vi "ACT_Loop.vi"() -> ()   [LabVIEW 2023, in "2024 Elevator_ACT.lvlib"]
uses:
  2024 Elevator_ACT.lvlib
  Cluster_CMD_ACT_Data.ctl
  <vilib>/Rock Robotics/WPI/Solenoid/WPI_SolenoidValue.ctl
  ENUM_ACT_State.ctl
  <vilib>/Rock Robotics/WPI/Compressor/WPI_CompressorDevRef.ctl
  <vilib>/Rock Robotics/WPI/Solenoid/WPI_SolenoidChannel.ctl
  <vilib>/Rock Robotics/WPI/Solenoid/WPI_SolenoidDevRef.ctl
  ENUM_ACT_Action.ctl
  <vilib>/Rock Robotics/WPI/Compressor/WPI_CompressorFeedbackMode.ctl
  <vilib>/Rock Robotics/WPI/Solenoid/WPI_SolenoidOpenDouble.vi
  RoboRIO Utilities/Global_STOP.vi
  Global_CMD_ACT_Data In.vi
  <vilib>/Rock Robotics/WPI/Solenoid/WPI_SolenoidSetEnum.vi
  Global_ACT_Data Out.vi
panel:
  out "Lift Output":T1
  out "Comp Enabled":bool
  out "Comp Running":bool
  out "Input DBL Data":T2
  out "Output DBL Data":dbl
  out "Cycle Time (S)":dbl format="%.3g"
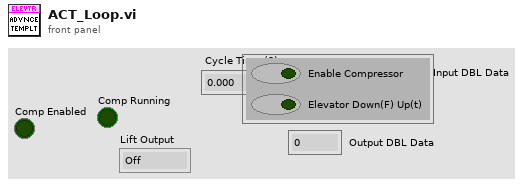
[diagram p1: front panel]
types:
  T1 = typedef "WPI_SolenoidValue.ctl" = enum16{"Off", "On", "Forward", "Reverse"}
  T2 = typedef "2024 Elevator_ACT.lvlib/Cluster_CMD_ACT_Data.ctl" = cluster{"Enable Compressor":bool, "Elevator Down(F) Up(t)":bool}
  T3 = typedef "WPI_SolenoidDevRef.ctl" = cluster{"DevStatus":errorcluster, "Pneumatics Control Module":u8, "Forward Solenoid Channel":T4, "Reverse Solenoid Channel":T4}
  T4 = typedef "WPI_SolenoidChannel.ctl" = enum8{"Solenoid 0", "Solenoid 1", "Solenoid 2", "Solenoid 3", "Solenoid 4", "Solenoid 5", "Solenoid 6", "Solenoid 7", "Solenoid 8", "Solenoid 9", "Solenoid 10", "Solenoid 11", "Solenoid 12", "Solenoid 13", "Solenoid 14", "Solenoid 15", "Invalid"}
  T5 = typedef "WPI_CompressorDevRef.ctl" = cluster{"DevStatus":errorcluster, "Pneumatics Control Module":u8}
  T6 = typedef "2024 Elevator_ACT.lvlib/ENUM_ACT_State.ctl" = enum16{"Startup", "Compressing", "NOT Compressing", "Shutdown"}
  T7 = cluster{"CompressorDevRef":T5, "State":T6, "Previous State":T6, "Current Time":timestamp, "Previous Time":timestamp, "Start Time":timestamp, "Target Time (ms)":u32, "Cycle Time(S)":dbl, "ACT Input":T2, "ACT Output DBL":dbl, "Elevator Ref":T3, "Previous CMD Elevator":bool, "ELEVATOR change":bool, "Comp Enabled":bool, "Comp Running":bool, "Lift Output":T1}
  T8 = typedef "WPI_CompressorFeedbackMode.ctl" = enum16{"Analog Only", "Digital Only", "Hybrid"}
  T9 = cluster{"Feedback Sensor":T8, "Max Pressure (PSI)":dbl, "Min Pressure (PSI)":dbl}
  T10 = typedef "2024 Elevator_ACT.lvlib/ENUM_ACT_Action.ctl" = enum16{"No Action", "Reset Time", "Reset All", "Start Compressor", "Stop Compressor", "Lift Solenoid", "Lower Solenoid", "OFF Solenoid"}
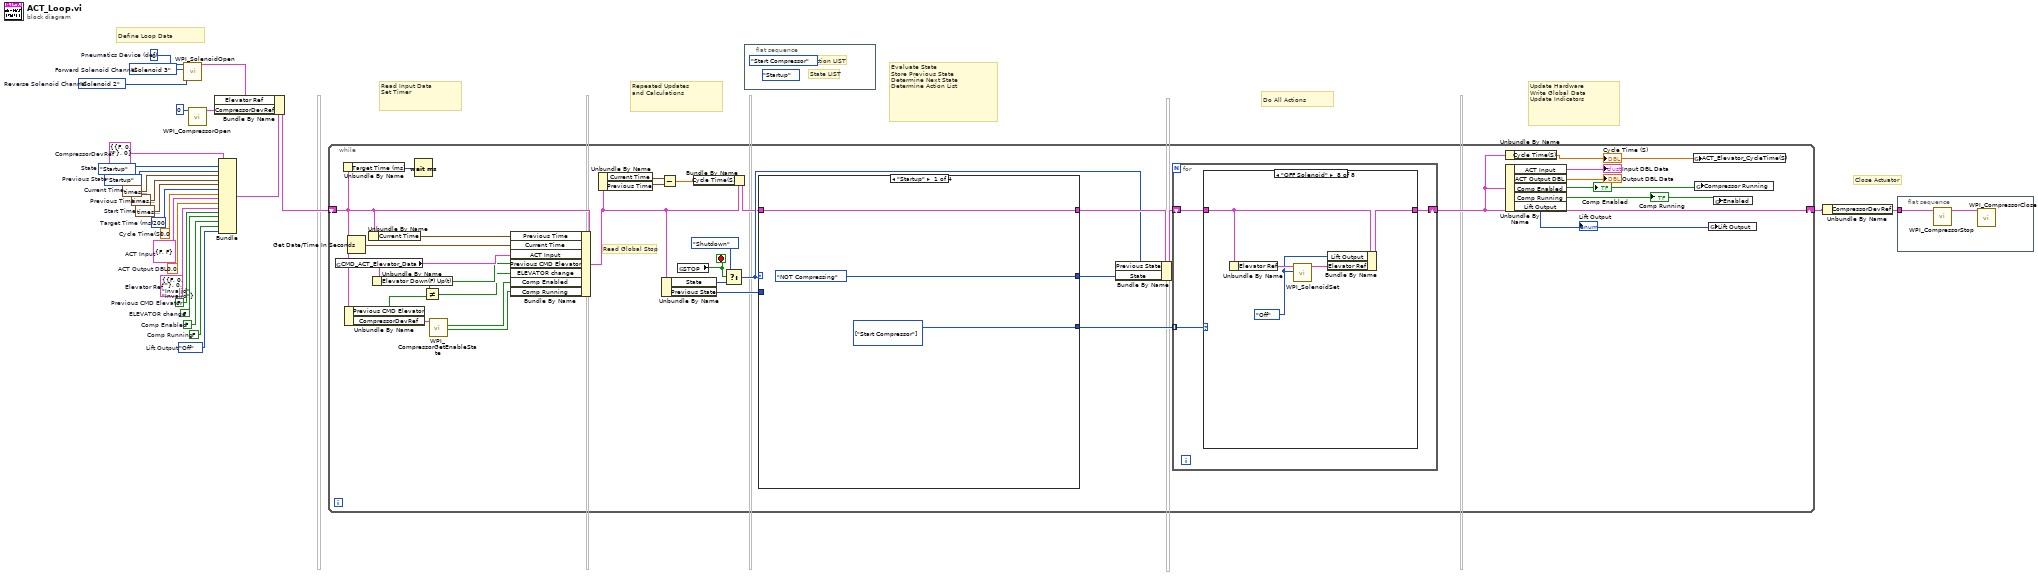
[diagram p0: block diagram]
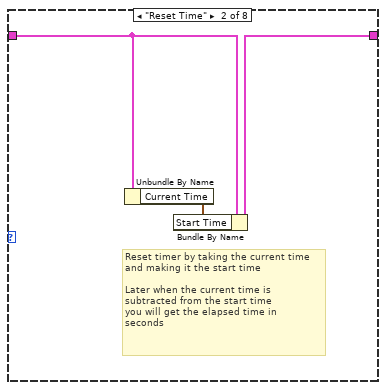
[diagram p3: hidden frame]
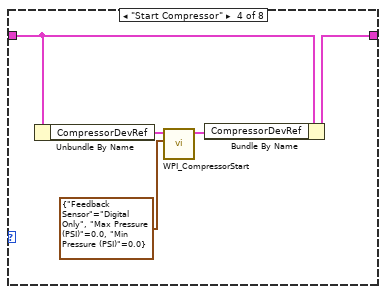
[diagram p5: hidden frame]
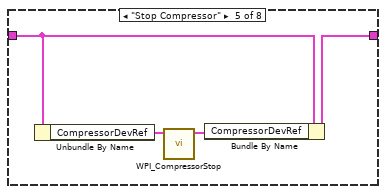
[diagram p6: hidden frame]
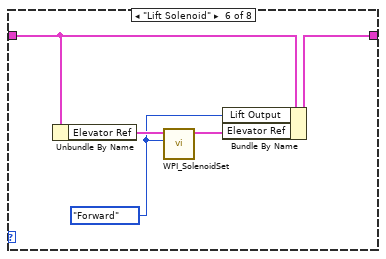
[diagram p7: hidden frame]
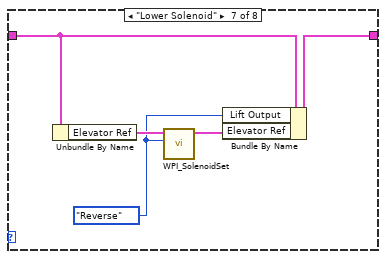
[diagram p8: hidden frame]
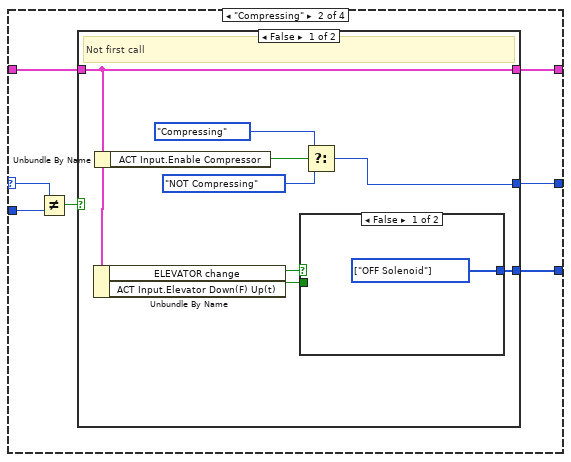
[diagram p9: hidden frame]
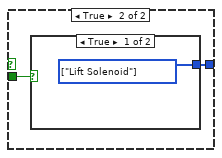
[diagram p10: hidden frame]
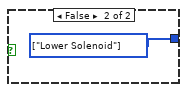
[diagram p11: hidden frame]
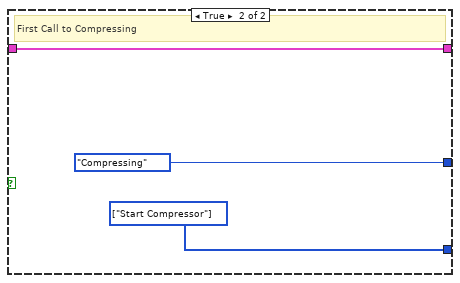
[diagram p12: hidden frame]
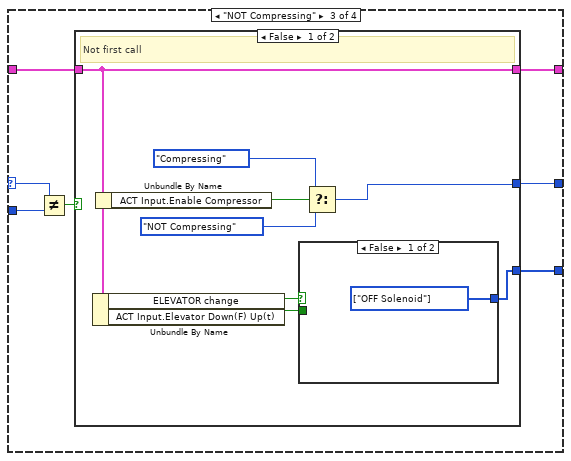
[diagram p13: hidden frame]
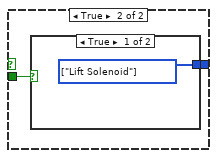
[diagram p14: hidden frame]
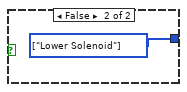
[diagram p15: hidden frame]
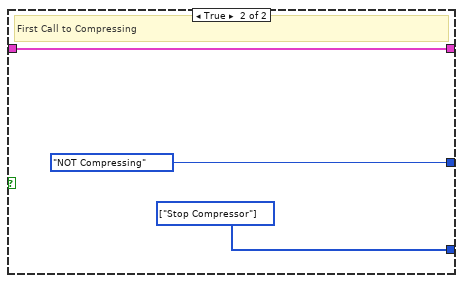
[diagram p16: hidden frame]
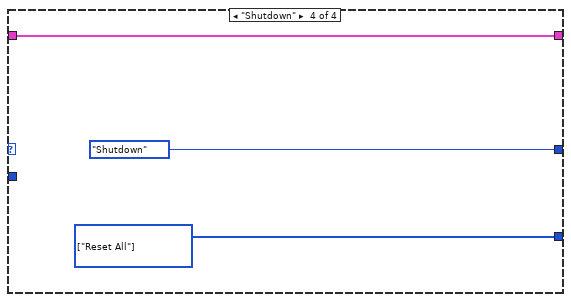
[diagram p17: hidden frame]
diagram:
  w1 = WPI_SolenoidValue."Off"  # Lift Output
  w2 = FALSE  # Comp Running
  w3 = FALSE  # Comp Enabled
  w4 = FALSE  # ELEVATOR change
  w5 = FALSE  # Previous CMD Elevator
  w7 = T3 {"DevStatus"={"status"=FALSE, "code"=0, "source"=""}, "Pneumatics Control Module"=0, "Forward Solenoid Channel"=enum."Invalid", "Reverse Solenoid Channel"=enum."Invalid"}  # Elevator Ref
  w8 = WPI_SolenoidChannel."Solenoid 2"  # Reverse Solenoid Channel
  w9 = WPI_SolenoidChannel."Solenoid 3"  # Forward Solenoid Channel
  w10 = u8 0  # Pneumatics Device (def)
  w12 = T5 {"DevStatus"={"status"=FALSE, "code"=0, "source"=""}, "Pneumatics Control Module"=0}  # CompressorDevRef
  w18 = 0.0  # Cycle Time(S)
  w19 = ENUM_ACT_State."Startup"  # Previous State
  w20 = timestamp(0 s since 1904-01-01)  # Previous Time
  w21 = u32 200  # Target Time (ms)
  w22 = 0.0  # ACT Output DBL
  w23 = T2 {"Enable Compressor"=FALSE, "Elevator Down(F) Up(t)"=FALSE}  # ACT Input
  w24 = timestamp(0 s since 1904-01-01)  # Start Time
  w25 = timestamp(0 s since 1904-01-01)  # Current Time
  w26 = ENUM_ACT_State."Startup"  # State
  # "Close Actuator"
  # "Define Loop Data"
  # "Repeated Updates\nand Calculations"
  # "Read Input Data\nSet Timer"
  # "Evaluate State\nStore Previous State\nDetermine Next State\nDetermine Action List"
  # "Do All Actions"
  # "Update Hardware\nWrite Global Data\nUpdate Indicators"
  n1 = call-poly <vilib>:"WPI_SolenoidOpen.vi"("Reverse Solenoid Channel"=w8, "Forward Solenoid Channel"=w9, "Pneumatics Device (def)"=w10) -> ("SolenoidDevRef"=w6:T3)  [unwired: 7 in, 1 out]
  n2 = call <vilib>:"WPI_CompressorOpen.vi"("Pneumatics device (def)"=u8 0) -> ("CompressorDevRef"=w13:T5)  [unwired: 13 in, 1 out]
  n3 = Bundle("CompressorDevRef"=w12, "State"=w26, "Previous State"=w19, "Current Time"=w25, "Previous Time"=w20, "Start Time"=w24, "Target Time (ms)"=w21, "Cycle Time(S)"=w18, "ACT Input"=w23, "ACT Output DBL"=w22, "Elevator Ref"=w7, "Previous CMD Elevator"=w5, "ELEVATOR change"=w4, "Comp Enabled"=w3, "Comp Running"=w2, "Lift Output"=w1) -> (w15:T7)  [unwired: 1 in]
  n4 = Bundle By Name(cluster=w15, "Elevator Ref"=w6, "CompressorDevRef"=w13) -> (w14:T7)
  n5 = while {
    shift-right: [w36] -> w16
    shift-left: w14 -> [w38]
    stop <- w54 stop-if-true
    # "Read Global Stop"
    n6 = global read "Global_CMD_ACT_Data In.vi" "CMD_ACT_Elevator_Data"() -> (w35:T2)
    n7 = Unbundle By Name(w38) -> ("Target Time (ms)"=w51:u32)
    n8 = Unbundle By Name(w38) -> ("Previous CMD Elevator"=w34:bool, "CompressorDevRef"=w37:T5)
    n9 = Get Date/Time In Seconds() -> (seconds since 1Jan1904=w58:timestamp)
    n10 = Unbundle By Name(w38) -> ("Current Time"=w50:timestamp)
    n11 = Unbundle By Name(w35) -> ("Elevator Down(F) Up(t)"=w33:bool)
    n12 = Wait (ms)(milliseconds to wait=w51) -> ()  [unwired: 1 out]
    n13 = Not Equal?(x=w33, y=w34) -> (x != y?=w32:bool)
    n14 = call <vilib>:"WPI_CompressorGetEnableState.vi"("CompressorDevRef"=w37) -> ("Compressor Running"=w30:bool, "Enabled"=w31:bool)  [unwired: 4 in, 5 out]
    n15 = Bundle By Name(cluster=w38, "Previous Time"=w50, "Current Time"=w58, "ACT Input"=w35, "Previous CMD Elevator"=w33, "ELEVATOR change"=w32, "Comp Enabled"=w31, "Comp Running"=w30) -> (w44:T7)
    n16 = Unbundle By Name(w44) -> ("Current Time"=w45:timestamp, "Previous Time"=w46:timestamp)
    n17 = Subtract(x=w45, y=w46) -> (x-y=w42:dbl)
    n18 = Unbundle By Name(w44) -> ("State"=w52:T6, "Previous State"=w49:T6)
    n19 = global read "Global_STOP.vi" "STOP"() -> (w54:bool)
    n20 = Bundle By Name(cluster=w44, "Cycle Time(S)"=w42) -> (w43:T7)
    n21 = Select(t=ENUM_ACT_State."Shutdown" ("State"), s=w54, f=w52) -> (s? t:f=w47:T6)
    n22 = case shown="\"Startup\"" w47 {
      selector: w47 -> [_ w98 w121 _]
      tunnel: w43 -> [w93 w96 w119 w142]
      tunnel: [w93 w95 w118 w142] -> w56
      tunnel: [ENUM_ACT_State."NOT Compressing" ("State") w100 w123 ENUM_ACT_State."Shutdown" ("State")] -> w55
      tunnel: [w92 w97 w120 w140] -> w41
      tunnel: w49 -> [_ w99 w122 _]
      frame "Startup" {
        w92 = T10[] [enum."Start Compressor"] items=["No Action", "Reset Time", "Reset All", "Start Compressor", "Stop Compressor", "Lift Solenoid", "Lower Solenoid", "OFF Solenoid"] ("Actions")
      }
      frame "Compressing" {
        n23 = Not Equal?(x=w98, y=w99) -> (x != y?=w94:bool)
        n24 = case shown="False" w94 {
          tunnel: [w106 ENUM_ACT_State."Compressing" ("State")] -> w100
          tunnel: [w103 w115] -> w97
          tunnel: w96 -> [w104 w114]
          tunnel: [w104 w114] -> w95
          frame False {
            # "Not first call"
            n25 = Unbundle By Name(w104) -> ("ELEVATOR change"=w101:bool, "ACT Input.Elevator Down(F) Up(t)"=w102:bool)
            n26 = Unbundle By Name(w104) -> ("ACT Input.Enable Compressor"=w108:bool)
            n27 = case shown="False" w101 {
              tunnel: [w109 w111] -> w103
              tunnel: w102 -> [_ w110]
              frame False {
                w109 = T10[] [enum."OFF Solenoid"] items=["No Action", "Reset Time", "Reset All", "Start Compressor", "Stop Compressor", "Lift Solenoid", "Lower Solenoid", "OFF Solenoid"] ("Actions")
              }
              frame True {
                n28 = case shown="True" w110 {
                  tunnel: [w112 w113] -> w111
                  frame True {
                    w112 = T10[] [enum."Lift Solenoid"] items=["No Action", "Reset Time", "Reset All", "Start Compressor", "Stop Compressor", "Lift Solenoid", "Lower Solenoid", "OFF Solenoid"] ("Actions")
                  }
                  frame False {
                    w113 = T10[] [enum."Lower Solenoid"] items=["No Action", "Reset Time", "Reset All", "Start Compressor", "Stop Compressor", "Lift Solenoid", "Lower Solenoid", "OFF Solenoid"] ("Actions")
                  }
                }
              }
            }
            n29 = Select(t=ENUM_ACT_State."Compressing" ("State"), s=w108, f=ENUM_ACT_State."NOT Compressing" ("State")) -> (s? t:f=w106:T6)
          }
          frame True {
            w115 = T10[] [enum."Start Compressor"] items=["No Action", "Reset Time", "Reset All", "Start Compressor", "Stop Compressor", "Lift Solenoid", "Lower Solenoid", "OFF Solenoid"] ("Actions")
            # "First Call to Compressing"
          }
        }
      }
      frame "NOT Compressing" {
        n30 = Not Equal?(x=w121, y=w122) -> (x != y?=w117:bool)
        n31 = case shown="False" w117 {
          tunnel: [w129 ENUM_ACT_State."NOT Compressing" ("State")] -> w123
          tunnel: [w124 w138] -> w120
          tunnel: w119 -> [w125 w137]
          tunnel: [w125 w137] -> w118
          frame False {
            # "Not first call"
            n32 = Unbundle By Name(w125) -> ("ELEVATOR change"=w126:bool, "ACT Input.Elevator Down(F) Up(t)"=w127:bool)
            n33 = Unbundle By Name(w125) -> ("ACT Input.Enable Compressor"=w131:bool)
            n34 = case shown="False" w126 {
              tunnel: [w132 w134] -> w124
              tunnel: w127 -> [_ w133]
              frame False {
                w132 = T10[] [enum."OFF Solenoid"] items=["No Action", "Reset Time", "Reset All", "Start Compressor", "Stop Compressor", "Lift Solenoid", "Lower Solenoid", "OFF Solenoid"] ("Actions")
              }
              frame True {
                n35 = case shown="True" w133 {
                  tunnel: [w135 w136] -> w134
                  frame True {
                    w135 = T10[] [enum."Lift Solenoid"] items=["No Action", "Reset Time", "Reset All", "Start Compressor", "Stop Compressor", "Lift Solenoid", "Lower Solenoid", "OFF Solenoid"] ("Actions")
                  }
                  frame False {
                    w136 = T10[] [enum."Lower Solenoid"] items=["No Action", "Reset Time", "Reset All", "Start Compressor", "Stop Compressor", "Lift Solenoid", "Lower Solenoid", "OFF Solenoid"] ("Actions")
                  }
                }
              }
            }
            n36 = Select(t=ENUM_ACT_State."Compressing" ("State"), s=w131, f=ENUM_ACT_State."NOT Compressing" ("State")) -> (s? t:f=w129:T6)
          }
          frame True {
            w138 = T10[] [enum."Stop Compressor"] items=["No Action", "Reset Time", "Reset All", "Start Compressor", "Stop Compressor", "Lift Solenoid", "Lower Solenoid", "OFF Solenoid"] ("Actions")
            # "First Call to Compressing"
          }
        }
      }
      frame "Shutdown" {
        w140 = T10[] [enum."Reset All"] items=["No Action", "Reset Time", "Reset All", "Start Compressor", "Stop Compressor", "Lift Solenoid", "Lower Solenoid", "OFF Solenoid"] ("Actions")
      }
    }
    n37 = Bundle By Name(cluster=w56, "Previous State"=w47, "State"=w55) -> (w57:T7)
    n38 = for {
      tunnel: w41 -> [w61] mode=indexing
      shift-right: [w60] -> w36
      shift-left: w57 -> [w59]
      n39 = case shown="\"OFF Solenoid\"" w61 {
        tunnel: w59 -> [w62 w65 w66 w71 w75 w80 w85 w90]
        tunnel: [w62 w64 w66 w70 w74 w79 w84 w89] -> w60
        frame "No Action" {
        }
        frame "Reset Time" {
          # "Reset timer by taking the current time\nand making it the start time\n\nLater when the current time is \nsubtracted from the start time\nyou will get the elapsed time in \nseconds"
          n40 = Unbundle By Name(w65) -> ("Current Time"=w63:timestamp)
          n41 = Bundle By Name(cluster=w65, "Start Time"=w63) -> (w64:T7)
        }
        frame "Reset All" {
        }
        frame "Start Compressor" {
          n42 = Unbundle By Name(w71) -> ("CompressorDevRef"=w69:T5)
          n43 = call <vilib>:"WPI_CompressorStart.vi"("Feedback Configuration"=T9 {"Feedback Sensor"=enum."Digital Only", "Max Pressure (PSI)"=0.0, "Min Pressure (PSI)"=0.0}, "CompressorDevRef"=w69) -> ("CompressorDevRef"=w68:T5)  [unwired: 8 in, 1 out]
          n44 = Bundle By Name(cluster=w71, "CompressorDevRef"=w68) -> (w70:T7)
        }
        frame "Stop Compressor" {
          n45 = Unbundle By Name(w75) -> ("CompressorDevRef"=w73:T5)
          n46 = call <vilib>:"WPI_CompressorStop.vi"("CompressorDevRef"=w73) -> ("CompressorDevRef"=w72:T5)  [unwired: 9 in, 1 out]
          n47 = Bundle By Name(cluster=w75, "CompressorDevRef"=w72) -> (w74:T7)
        }
        frame "Lift Solenoid" {
          w76 = WPI_SolenoidValue."Forward" ("Value")
          n48 = Unbundle By Name(w80) -> ("Elevator Ref"=w78:T3)
          n49 = call-poly <vilib>:"WPI_SolenoidSet.vi"("Value"=w76, "SolenoidDevRef"=w78) -> ("SolenoidDevRef"=w77:T3)  [unwired: 8 in, 1 out]
          n50 = Bundle By Name(cluster=w80, "Lift Output"=w76, "Elevator Ref"=w77) -> (w79:T7)
        }
        frame "Lower Solenoid" {
          w81 = WPI_SolenoidValue."Reverse" ("Value")
          n51 = Unbundle By Name(w85) -> ("Elevator Ref"=w83:T3)
          n52 = call-poly <vilib>:"WPI_SolenoidSet.vi"("Value"=w81, "SolenoidDevRef"=w83) -> ("SolenoidDevRef"=w82:T3)  [unwired: 8 in, 1 out]
          n53 = Bundle By Name(cluster=w85, "Lift Output"=w81, "Elevator Ref"=w82) -> (w84:T7)
        }
        frame "OFF Solenoid" {
          w86 = WPI_SolenoidValue."Off" ("Value")
          n54 = Unbundle By Name(w90) -> ("Elevator Ref"=w88:T3)
          n55 = call-poly <vilib>:"WPI_SolenoidSet.vi"("Value"=w86, "SolenoidDevRef"=w88) -> ("SolenoidDevRef"=w87:T3)  [unwired: 8 in, 1 out]
          n56 = Bundle By Name(cluster=w90, "Lift Output"=w86, "Elevator Ref"=w87) -> (w89:T7)
        }
      }
    }
    n57 = Unbundle By Name(w36) -> ("Cycle Time(S)"=w39:dbl)
    "Cycle Time (S)" <- w39
    n58 = Unbundle By Name(w36) -> ("ACT Input"=→"Input DBL Data":T2, "ACT Output DBL"=→"Output DBL Data":dbl, "Comp Enabled"=w29:bool, "Comp Running"=w28:bool, "Lift Output"=w27:T1)
    "Comp Running" <- w28
    "Comp Enabled" <- w29
    "Lift Output" <- w27
    n59 = global write "Global_ACT_Data Out.vi" "ACT_Elevator_CycleTime(S)"(w39) -> ()
    n60 = global write "Global_ACT_Data Out.vi" "Compressor Running"(w29) -> ()
    n61 = global write "Global_ACT_Data Out.vi" "Lift Output"(w27) -> ()
    n62 = global write "Global_ACT_Data Out.vi" "Enabled"(w28) -> ()
  }
  n63 = flat-sequence {
    frame #0 {
      (unwired) ENUM_ACT_State."Startup" ("State")
      (unwired) ENUM_ACT_Action."Start Compressor" ("Action")
      # "State LIST"
      # "Action LIST"
    }
  }
  n64 = Unbundle By Name(w16) -> ("CompressorDevRef"=w17:T5)
  n65 = flat-sequence {
    tunnel: w17 -> [w143]
    frame #0 {
      n66 = call <vilib>:"WPI_CompressorStop.vi"("CompressorDevRef"=w143) -> ("CompressorDevRef"=w144:T5)  [unwired: 9 in, 1 out]
      n67 = call <vilib>:"WPI_CompressorClose.vi"("CompressorDevRef"=w144) -> ()  [unwired: 10 in, 1 out]
    }
  }
